vi "Queue Last Ack.vi"(10 "Queue Actor":refnum<class "Queue Actor.lvclass">, 11 "Hello World Queue in":refnum<class "Hello World Queue.lvclass">) -> (3 "Hello World Queue out":refnum<class "Hello World Queue.lvclass">)   [LabVIEW 2021, in "Hello World Queue.lvlib" / "Hello World Queue.lvclass"]
uses:
  Hello World Queue.lvclass
  jettl/Queue Actor/Queue Actor.lvclass
  Hello World Queue.lvclass/Hello World Queue.ctl
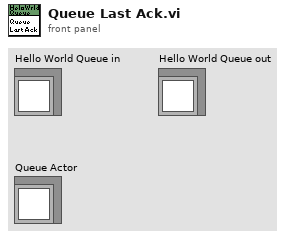
[diagram p1: front panel]
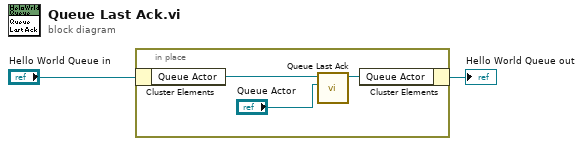
[diagram p0: block diagram]
diagram:
  n1 = in-place {
    n2 = in-place-cluster #1("Hello World Queue in") -> ("Queue Actor"=w5:refnum<class "Queue Actor.lvclass">)
    n3 = call-dynamic "Queue Last Ack.vi"("Queue Actor"="Queue Actor", "Queue Last Ack in"=w5) -> ("Queue Last Ack out"=w4:refnum<class "Queue Actor.lvclass">)  [unwired: 9 in]
    n4 = in-place-cluster #1("Queue Actor"=w4) -> (→"Hello World Queue out":refnum<class "Hello World Queue.lvclass">)
  }
